vi "ACC_LabVIEW_VI-Tree.vi"   [LabVIEW 2014, in "ACC_LabVIEW.lvlib"]
doc: "License Agreement for this software:\n\nCopyright (C)\nGesellschaft für Schwerionenforschung, GSI\nPlanckstr. 1\n64291 Darmstadt\nGermany\n\nContact: al.schwinn@gsi.de\n\nThis program is free software; you can redistribute it and/or modify it under the terms of the \nGNU General Public License as published by the Free Software Foundation; either version 2 of \nthe license, or (at your option) any later version.\n\nThis program is distributed in the hope that it will be useful, but WITHOUT ANY WARRANTY; \nwithout even the implied warranty of MERCHANTABILITY or FITNESS FOR A PARTICULAR PURPOSE. See the GNU General License for more details (http://www.gnu.org).\n\nGesellschaft für Schwerionenforschung, GSI\nPlanckstr. 1, 64291 Darmstadt, Germany\nFor all questions and ideas contact: al.schwinn@gsi.de or H.Brand@gsi.de or D.Beck@gsi.de.\nLast update: 24-OKT-2008"
uses:
  ACC_LabVIEW.lvlib
  DataConverter/LabVIEW2AccData_Float64.vi
  DataConverter/Acc2LabVIEWData_Float64.vi
panel:
  # "Refer to blockdiagram."
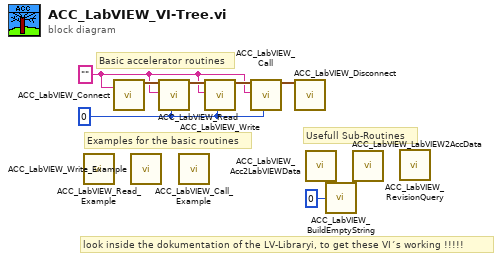
[diagram p0: block diagram]
diagram:
  w1 = "" ("Nomenklatur")
  w7 = 0
  # "look inside the dokumentation of the LV-Libraryi, to get these VI´s working !!!!!"
  # "Usefull Sub-Routines"
  # "Examples for the basic routines"
  # "Basic accelerator routines"
  n1 = call "ACC_LabVIEW_Read_Example.vi"() -> ()  [unwired: 12 in]
  n2 = call "ACC_LabVIEW_Connect.vi"("Nomenklatur"=w1) -> ("DeviceReferenceOut"=w3:cluster{"ID":u32})  [unwired: 17 in, 1 out]
  n3 = call "ACC_LabVIEW_Write_Example.vi"() -> ()  [unwired: 1 in]
  n4 = call "ACC_LabVIEW_Read.vi"("DeviceReferenceIn"=w3, "Propname"=w1, "VirtAcc"=w7) -> ("DeviceReferenceOut"=w5:cluster{"ID":u32})  [unwired: 12 in, 4 out]
  n5 = call "ACC_LabVIEW_Call_Example.vi"() -> ()  [unwired: 20 in]
  n6 = call "ACC_LabVIEW_Write.vi"("DeviceReferenceIn"=w5, "Propname"=w1, "VirtAcc"=w7) -> ("DeviceReferenceOut"=w4:cluster{"ID":u32})  [unwired: 14 in, 2 out]
  n7 = call "ACC_LabVIEW_Call.vi"("DeviceReferenceIn"=w4, "Propname"=w1, "VirtAcc"=w7) -> ("DeviceReferenceOut"=w2:cluster{"ID":u32})  [unwired: 15 in, 1 out]
  n8 = call "ACC_LabVIEW_Disconnect.vi"("DeviceReferenceIn"=w2) -> ()  [unwired: 18 in, 1 out]
  n9 = call-poly "ACC_LabVIEW_Acc2LabVIEWData.vi"() -> ()  [unwired: 17 in, 3 out]
  n10 = call "ACC_LabVIEW_BuildEmptyString.vi"("Length"=u32 0) -> ()  [unwired: 1 out]
  n11 = call-poly "ACC_LabVIEW_LabVIEW2AccData.vi"() -> ()  [unwired: 19 in, 1 out]
  n12 = call "ACC_LabVIEW_RevisionQuery.vi"() -> ()  [unwired: 2 out]
